vi "MLUG_SpecPage.vi"(10 "Spec Page Interface":T1, 11 "MetaDataObj in":refnum<class "MetaDataObj.lvclass">) -> (3 "MetaDataObj out":refnum<class "MetaDataObj.lvclass">)   [LabVIEW 2020, in "MLUG.lvclass"]
uses:
  MLUG.lvclass
  MLUG.lvclass/MLUG.ctl
  C:/Program Files (x86)/National Instruments/LabVIEW 2020/resource/dialog/NewProjectWizard/MetaDataObj/MetaDataObj.lvclass
  C:/Program Files (x86)/National Instruments/LabVIEW 2020/ProjectTemplates/Source/MLUG/scripting/MLUG/MLUG.lvclass
  <resource>/dialog/NewProjectWizard/Spec Page Interface.ctl
  <resource>/dialog/NewProjectWizard/MetaDataObj/MetaDataObj.lvclass
panel:
  in  "Project Name":string
  in  "Project Root":path
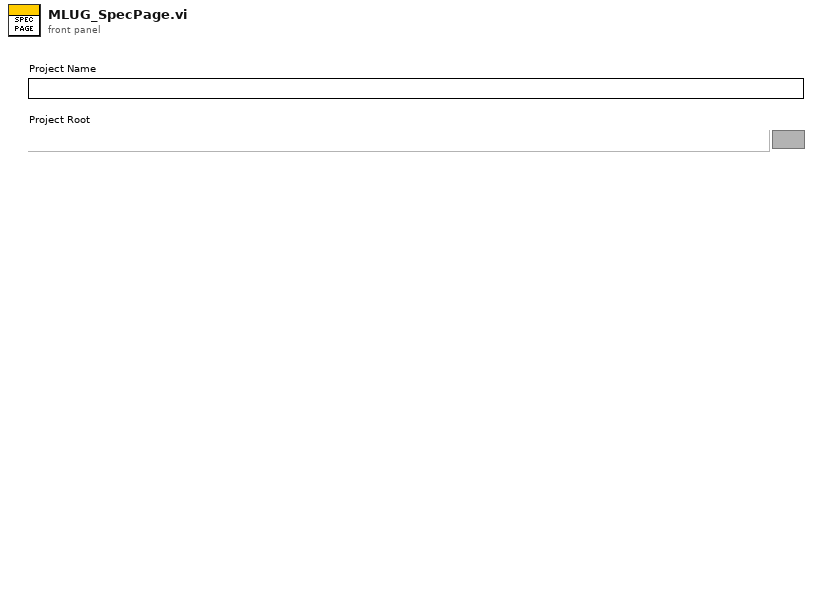
[diagram p1: front panel]
types:
  T1 = typedef "Spec Page Interface.ctl" = cluster{"\"Tab Forward To\" Refnum":refnum<vi>, "\"Tab Backward To\" Refnum":refnum<vi>, "Errors":refnum<user-event>, "Quit":refnum<user-event>}
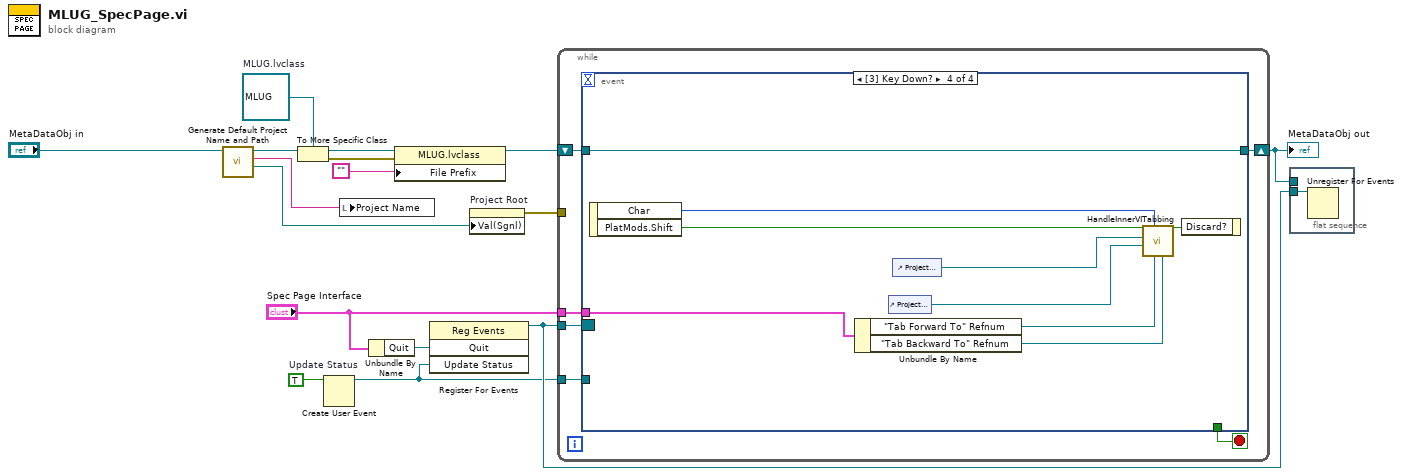
[diagram p0: block diagram]
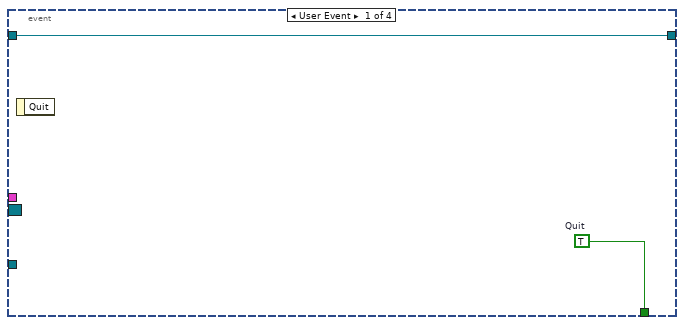
[diagram p2: hidden frame]
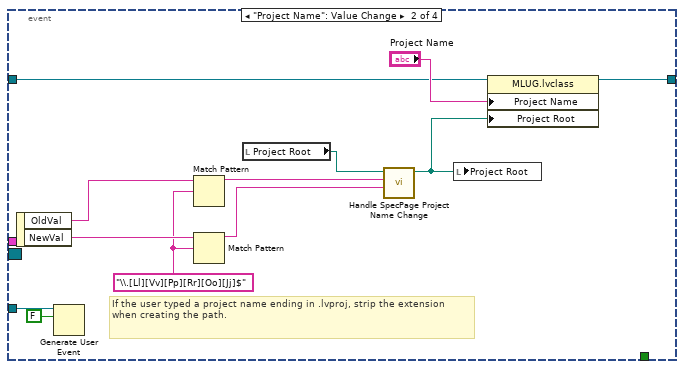
[diagram p3: hidden frame]
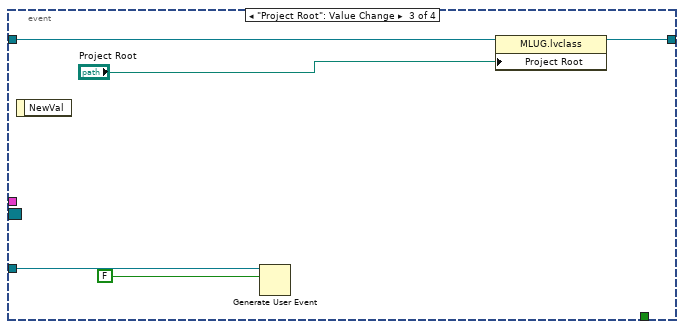
[diagram p4: hidden frame]
diagram:
  w1 = refnum<class "MLUG.lvclass"> refnum  # MLUG.lvclass
  w11 = TRUE  # Update Status
  n1 = call <resource>:"Generate Default Project Name and Path.vi"("DNL_MetaDataObj in"="MetaDataObj in") -> ("Project Root"=w3:path, "Project Name"=w2:string, "DNL_MetaDataObj out"=w4:refnum<class "MetaDataObj.lvclass">)  [unwired: 8 in]
  n2 = To More Specific Class(target class=w1, reference=w4) -> (specific class reference=w13:refnum<class "MLUG.lvclass">, error out=w12:errorcluster)  [unwired: 1 in]
  n3 = Create User Event(user event datatype=w11) -> (user event=w8:refnum<user-event>)  [unwired: 1 in, 1 out]
  n4 = local write "Project Name"(w2) -> ()
  n5 = Unbundle By Name("Spec Page Interface") -> ("Quit"=w16:refnum<user-event>)
  n6 = property class="MLUG.lvclass"(reference=w13, error in=w12, "File Prefix"="") -> (reference out=w10:refnum<class "MLUG.lvclass">)  [unwired: 1 out]
  n7 = register-events(w16, w8) -> (reference out=w15:refnum<event-registration>)  [unwired: 2 in, 1 out]
  n8 = property on="Project Root" class="Path"("Val(Sgnl)"=w3) -> (error out=w9:errorcluster)  [unwired: 2 in, 1 out]
  n9 = while {
    tunnel: "Spec Page Interface" -> [w21]
    shift-right: [w19] -> w6
    shift-left: w10 -> [w18]
    tunnel: w15 -> [w20]
    tunnel: w9 -> [_]
    tunnel: w8 -> [w17]
    stop <- w22 stop-if-true
    n10 = event shown="[3] Key Down?" {
      selector: w20 -> [_ _ _ _]
      dyn-events: _ -> [_ _ _ _]
      timeout: _ -> [_ _ _ _]
      tunnel: w21 -> [_ _ _ w46]
      tunnel: [w24 _ _ _] -> w22
      tunnel: [w23 w36 w40 w43] -> w19
      tunnel: w18 -> [w23 w32 w41 w43]
      tunnel: w17 -> [_ w35 w39 _]
      event User Event {
        w24 = TRUE  # Quit
        n11 = event-data() -> ()  [unwired: 1 in, 1 out]
      }
      event "Project Name": Value Change {
        w27 = "\\.[Ll][Vv][Pp][Rr][Oo][Jj]$" ("regular expression")
        # "If the user typed a project name ending in .lvproj, strip the extension when creating the path."
        n12 = event-data() -> ("OldVal"=w29:string, "NewVal"=w28:string)  [unwired: 1 in]
        n13 = Generate User Event(user event=w35, event data cluster=FALSE ("Update Status")) -> ()  [unwired: 2 in, 2 out]
        n14 = Match Pattern(string=w29, regular expression=w27) -> (before substring=w26:string)  [unwired: 1 in, 3 out]
        n15 = Match Pattern(string=w28, regular expression=w27) -> (before substring=w25:string)  [unwired: 1 in, 3 out]
        n16 = local read "Project Root"() -> (w31:path)
        n17 = call <resource>:"Handle SpecPage Project Name Change.vi"("Project Name New Value"=w25, "Project Name Old Value"=w26, "Project Root in"=w31) -> ("Project Root out"=w30:path)  [unwired: 8 in]
        n18 = local write "Project Root"(w30) -> ()
        n19 = property class="MLUG.lvclass"(reference=w32, "Project Name"="Project Name", "Project Root"=w30) -> (reference out=w36:refnum<class "MLUG.lvclass">)  [unwired: 1 in, 1 out]
      }
      event "Project Root": Value Change {
        n20 = event-data() -> ()  [unwired: 1 in, 1 out]
        n21 = Generate User Event(user event=w39, event data cluster=FALSE ("Update Status")) -> ()  [unwired: 2 in, 2 out]
        n22 = property class="MLUG.lvclass"(reference=w41, "Project Root"="Project Root") -> (reference out=w40:refnum<class "MLUG.lvclass">)  [unwired: 1 in, 1 out]
      }
      event Key Down? {
        n23 = event-data() -> ("Char"=w49:i16, "PlatMods.Shift"=w48:bool)  [unwired: 1 in]
        n24 = Unbundle By Name(w46) -> ("\"Tab Forward To\" Refnum"=w45:refnum<vi>, "\"Tab Backward To\" Refnum"=w44:refnum<vi>)
        n25 = control-ref of="Project Root"() -> (w42:refnum<vi>)
        n26 = control-ref of="Project Name"() -> (w47:refnum<vi>)
        n27 = call <resource>:"HandleInnerVITabbing.vi"("Tab Backward To"=w44, "Tab Forward To"=w45, "Char"=w49, "Last Control"=w42, "First Control"=w47, "Shift"=w48) -> ("Discard"=w50:bool)  [unwired: 5 in]
        n28 = event-data("Discard?"=w50) -> ()  [unwired: 1 in, 1 out]
      }
    }
  }
  "MetaDataObj out" <- w6
  n29 = flat-sequence {
    tunnel: w15 -> [w51]
    tunnel: w6 -> [_]
    frame #0 {
      n30 = Unregister For Events(event registration refnum=w51) -> ()  [unwired: 1 in, 1 out]
    }
  }
